vi "lectura.vi"(9 "Numeric in":i32, 10 "Numeric 3":i32, 11 "entrada1":i32) -> (1 "Numeric 4":i32, 2 "Real Matrix Element 2":dbl, 3 "salida1":i32, 4 "Numeric out":i32, 5 "Real Matrix Element 3":dbl, 6 "Real Matrix Element":dbl)   [LabVIEW 2017]
uses:
  <vilib>/Analysis/Matrix/Datatypes/RealMatrix.ctl
  <vilib>/Analysis/Matrix/NI_Matrix.lvlib
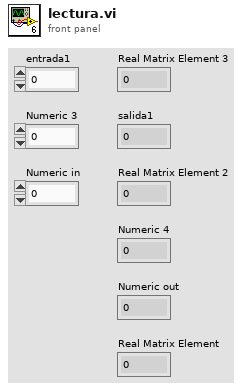
[diagram p1: front panel]
types:
  T1 = typedef "NI_Matrix.lvlib/RealMatrix.ctl" = dbl[][]
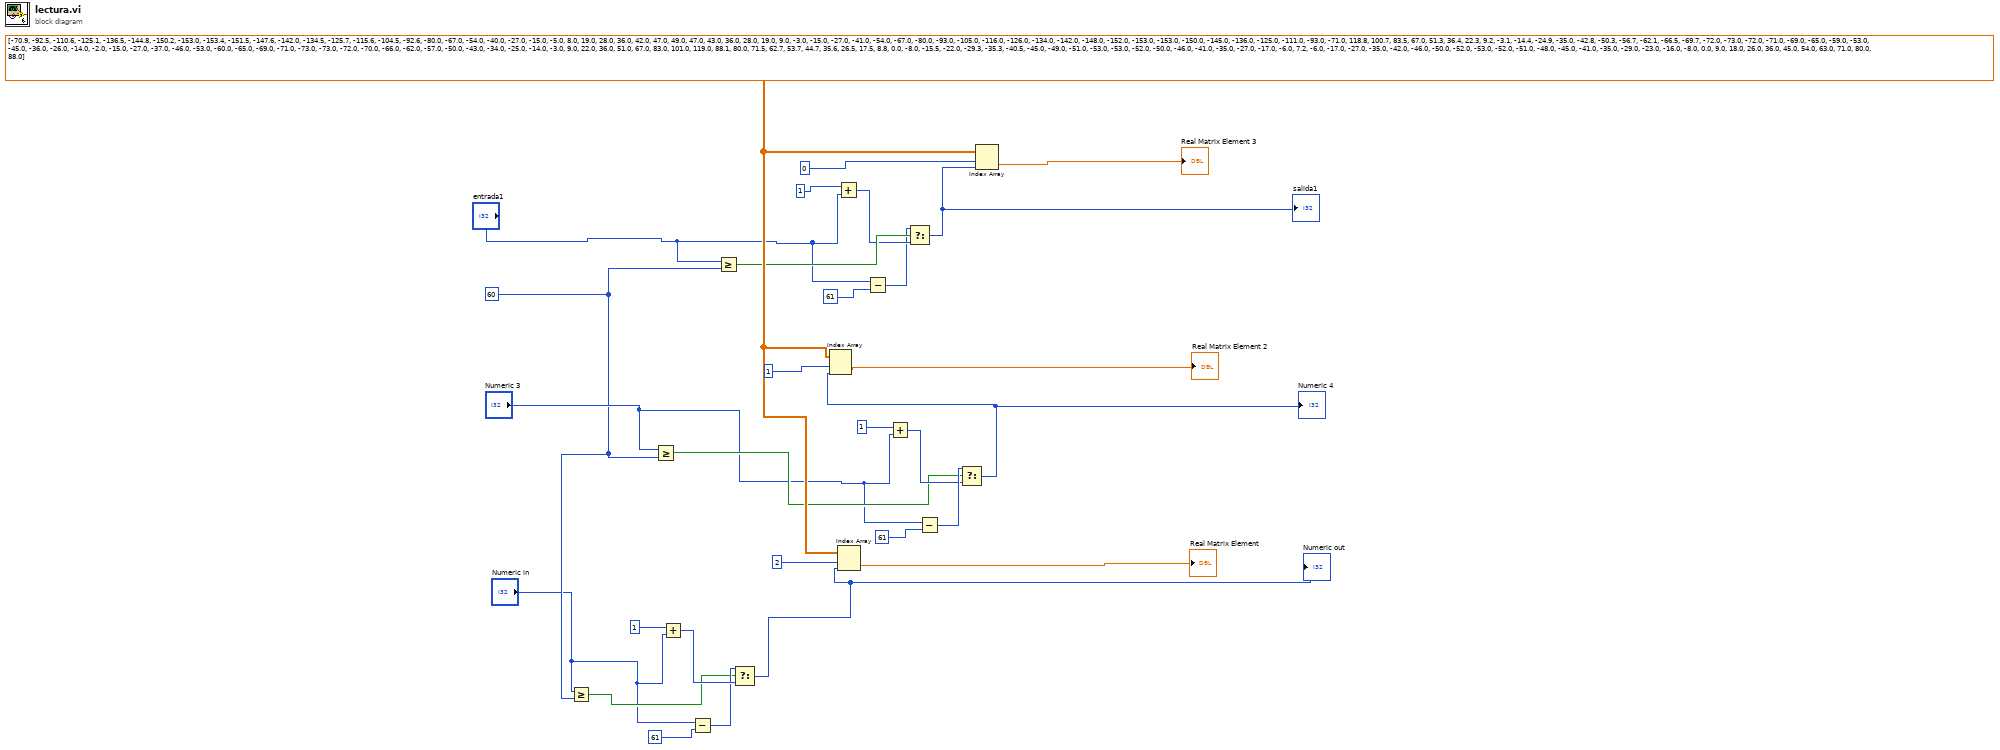
[diagram p0: block diagram]
diagram:
  w3 = 60 ("y")
  w26 = T1 [[-70.9, -92.5, -110.6, -125.1, -136.5, -144.8, -150.2, -153.0, -153.4, -151.5, -147.6, -142.0, -134.5, -125.7, -115.6, -104.5, -92.6, -80.0, -67.0, -54.0, -40.0, -27.0, -15.0, -5.0, 8.0, 19.0, 28.0, 36.0, 42.0, 47.0, 49.0, 47.0, 43.0, 36.0, 28.0, 19.0, 9.0, -3.0, -15.0, -27.0, -41.0, -54.0, -67.0, -80.0, -93.0, -105.0, -116.0, -126.0, -134.0, -142.0, -148.0, -152.0, -153.0, -153.0, -150.0, -145.0, -136.0, -125.0, -111.0, -93.0, -71.0], [118.8, 100.7, 83.5, 67.0, 51.3, 36.4, 22.3, 9.2, -3.1, -14.4, -24.9, -35.0, -42.8, -50.3, -56.7, -62.1, -66.5, -69.7, -72.0, -73.0, -72.0, -71.0, -69.0, -65.0, -59.0, -53.0, -45.0, -36.0, -26.0, -14.0, -2.0, -15.0, -27.0, -37.0, -46.0, -53.0, -60.0, -65.0, -69.0, -71.0, -73.0, -73.0, -72.0, -70.0, -66.0, -62.0, -57.0, -50.0, -43.0, -34.0, -25.0, -14.0, -3.0, 9.0, 22.0, 36.0, 51.0, 67.0, 83.0, 101.0, 119.0], [88.1, 80.0, 71.5, 62.7, 53.7, 44.7, 35.6, 26.5, 17.5, 8.8, 0.0, -8.0, -15.5, -22.0, -29.3, -35.3, -40.5, -45.0, -49.0, -51.0, -53.0, -53.0, -52.0, -50.0, -46.0, -41.0, -35.0, -27.0, -17.0, -6.0, 7.2, -6.0, -17.0, -27.0, -35.0, -42.0, -46.0, -50.0, -52.0, -53.0, -52.0, -51.0, -48.0, -45.0, -41.0, -35.0, -29.0, -23.0, -16.0, -8.0, 0.0, 9.0, 18.0, 26.0, 36.0, 45.0, 54.0, 63.0, 71.0, 80.0, 88.0]] ("matrix")
  n1 = Greater Or Equal?(x="Numeric in", y=w3) -> (x >= y?=w4:bool)
  n2 = Greater Or Equal?(x="Numeric 3", y=w3) -> (x >= y?=w11:bool)
  n3 = Add(x=1 ("index (col)"), y="Numeric in") -> (x+y=w7:i32)
  n4 = Subtract(x="Numeric in", y=61) -> (x-y=w6:i32)
  n5 = Greater Or Equal?(x="entrada1", y=w3) -> (x >= y?=w21:bool)
  n6 = Select(t=w6, s=w4, f=w7) -> (s? t:f=w5:i32)
  "Numeric out" <- w5
  n7 = Add(x=1 ("index (col)"), y="entrada1") -> (x+y=w20:i32)
  n8 = Index Array(array=w26, index (row)=2, index (col)=w5) -> (element=→"Real Matrix Element":dbl)
  n9 = Subtract(x="entrada1", y=61) -> (x-y=w18:i32)
  n10 = Add(x=1 ("index (col)"), y="Numeric 3") -> (x+y=w13:i32)
  n11 = Select(t=w18, s=w21, f=w20) -> (s? t:f=w19:i32)
  "salida1" <- w19
  n12 = Subtract(x="Numeric 3", y=61) -> (x-y=w14:i32)
  n13 = Select(t=w14, s=w11, f=w13) -> (s? t:f=w9:i32)
  "Numeric 4" <- w9
  n14 = Index Array(array=w26, index (row)=1, index (col)=w9) -> (element=→"Real Matrix Element 2":dbl)
  n15 = Index Array(array=w26, index (row)=0, index (col)=w19) -> (element=→"Real Matrix Element 3":dbl)
